vi "OE1022D_Configure Sensitivity and Filter.vi"(7 "OE1022D_Configure Sens and Filter":T1={"Dynamic Reserve"=1, "Sensitivity "=24, "Time Constant "=9, "Low Pass Filter Slope "=1, "Enable Sync Filter"=0, "Channel"=1} {"Channel" items=["A"=1, "B"=2]; "Enable Sync Filter" items=["OFF", "ON"]; "Low Pass Filter Slope" items=["6 dB/oct", "12 dB/oct", "18 db/oct", "24 dB/oct"]; "Time Constant" items=["10 us", "30 us", "100 us", "300 us", "1 ms", "3 ms", "10 ms", "30 ms", "100 ms", "300 ms", "1 s", "3 s", "10 s", "30 s", "100 s", "300 s", "1 ks", "3 ks"]; "Sensitivity" items=["1 nV/fA", "2 nV/fA", "5 nV/fA", "10 nV/fA", "20 nV/fA", "50 nV/fA", "100 nV/fA", "200 nV/fA", "500 nV/fA", "1 uV/pA", "2 uV/pA", "5 uV/pA", "10 uV/pA", "20 uV/pA", "50 uV/pA", "100 uV/pA", "200 uV/pA", "500 uV/pA", "1 mV/nA", "2 mV/nA", "5 mV/nA", "10 mV/nA", "20 mV/nA", "50 mV/nA", "100 mV/nA", "200 mV/nA", "500 mV/nA", "1 V/uA"]; "Dynamic Reserve" items=["Low Noise", "Normal", "High Reserve"]}, 8 "Error in (no error)":errorcluster caption="error out（no error）", 9 "Remote Mode":u16(ring) items=["USB", "RS232", "GPIB"], 11 "VISA resource name":refnum<visa-resource-name>) -> (0 "Error out":errorcluster caption="error out", 1 "Output String":string, 3 "VISA resource  out":refnum<visa-resource-name>)   [LabVIEW 2011]
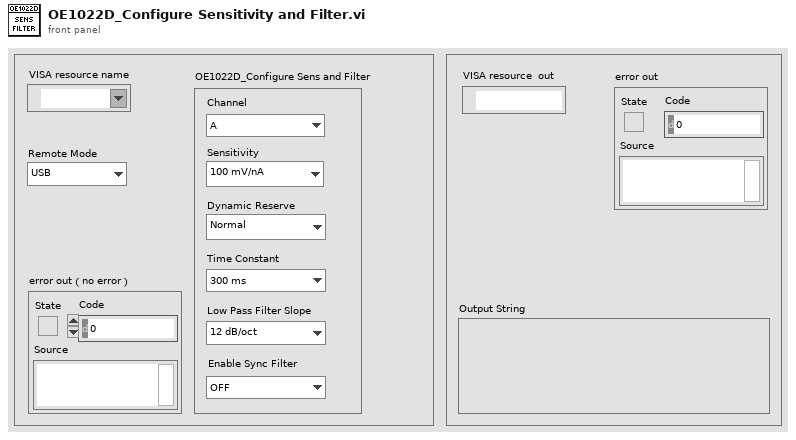
[diagram p1: front panel]
types:
  T1 = cluster{"Dynamic Reserve":u16, "Sensitivity ":u16, "Time Constant ":u8, "Low Pass Filter Slope ":u8, "Enable Sync Filter":u16, "Channel":u16}
  T2 = enum16{"ISRC", "IGND", "ICPL", "ILIN", "PHAS", "FMOD", "RSLP", "FREQ", "SWPT", "SLLM", "SULM", "SSLL", "SSLG", "STLM", "SWRM", "IRNG", "SENS", "RMOD", "OFLT", "OFSL", "SYNC", "DMOD", "HARM", "DARB", "SWVT", "SLVL", "SVLL", "SVUL", "SVSL", "SVSG", "SVTM", "SVRM", "RALL", "SNAP", "OUTP", "OAUX", "COUT", "CAUX", "COFP", "CEXP", "FPOP", "OEXP", "*IDN", "*RST", "OVLD", "INOV", "GNOV", "*PLL", "SSET", "RSET", "AGAN", "APHS", "ARSV", "ASCL", "EQCD", "EQCS", "SPED", "SRAT", "SLEN", "SSLE", "STRG", "SPRM", "STRD", "PAUS", "REST", "SPTS", "TRCA", "TEMP", "RSTU", "IHNZ", "DEQU", "SADD", "ARNG", "CSPE", "ISRCD", "IGNDD", "ICPLD", "ILIND", "PHASD", "FMODD", "RSLPD", "FREQD", "SWPTD", "SLLMD", "SULMD", "SSLLD", "SSLGD", "STLMD", "SWRMD", "SENSD", "RMODD", "OFLTD", "OFSLD", "SYNCD", "HARMD", "EQCDD", "EQCSD", "SNAPD", "OUTPD", "SWVTD", "SLVLD", "SVLLD", "SVULD", "SVSLD", "SVSGD", "SVTMD", "SVRMD", "SVDCD", "ARSVD", "AGAND", "APHSD", "ASCLD", "FPOPD", "CAUXD", "OEXPD", "SPEDD", "SRATD", "SLEND", "SSLED", "STRGD", "SPRMD", "STRDD", "PAUSD", "RESTD", "SPTSD", "TRCAD", "*IDND", "*RSTD", "INOVD", "GNOVD", "*PLLD", "SSETD", "RSETD"}
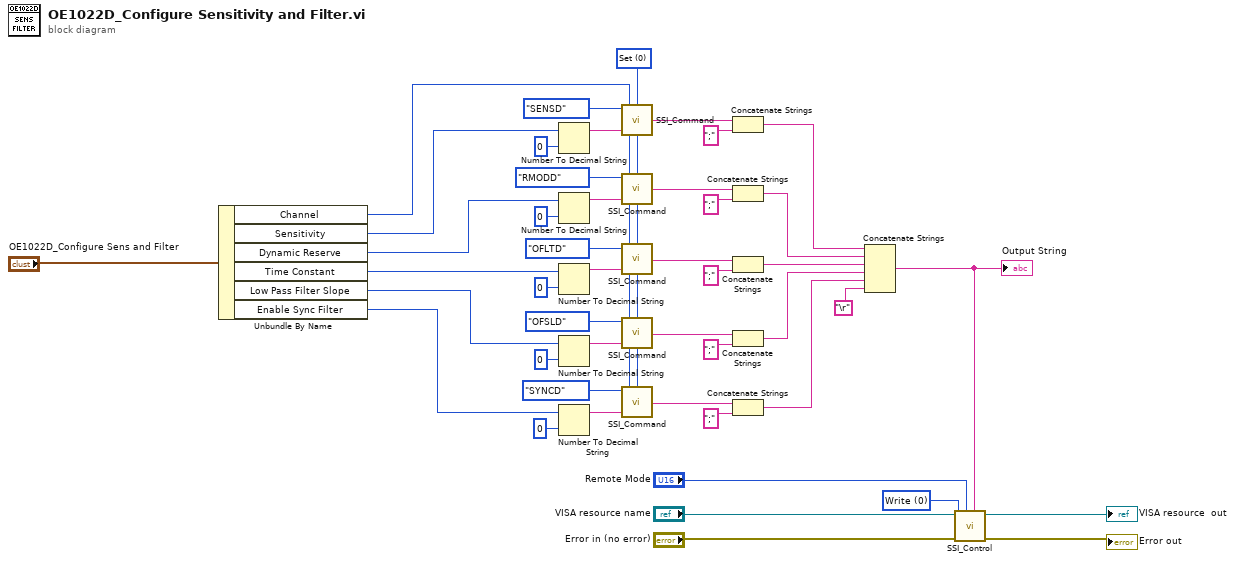
[diagram p0: block diagram]
diagram:
  w11 = u16 0 items=["Set", "Query"] ("Opera")
  w45 = u16 0 items=["Write", "Read"] ("Control")
  n1 = Unbundle By Name("OE1022D_Configure Sens and Filter") -> ("Channel"=w3:u16, "Sensitivity"=w21:u16, "Dynamic Reserve"=w20:u16, "Time Constant"=w19:u8, "Low Pass Filter Slope"=w18:u8, "Enable Sync Filter"=w10:u16)
  n2 = Number To Decimal String(number=w21, width (-)=i16 0 ("精度(6)")) -> (decimal integer string=w40:string)
  n3 = Number To Decimal String(number=w20, width (-)=i16 0 ("宽度(-)")) -> (decimal integer string=w38:string)
  n4 = Number To Decimal String(number=w19, width (-)=i16 0 ("宽度(-)")) -> (decimal integer string=w36:string)
  n5 = Number To Decimal String(number=w18, width (-)=i16 0 ("精度(6)")) -> (decimal integer string=w34:string)
  n6 = Number To Decimal String(number=w10, width (-)=i16 0 ("精度(6)")) -> (decimal integer string=w15:string)
  n7 = call "SSI_Command.vi"("Opera"=w11, "Paramter"=w40, "channel"=w3, "Command Type"=T2."SENSD") -> ("Output string"=w27:string)
  n8 = call "SSI_Command.vi"("Opera"=w11, "Paramter"=w38, "channel"=w3, "Command Type"=T2."RMODD") -> ("Output string"=w31:string)
  n9 = call "SSI_Command.vi"("Opera"=w11, "Paramter"=w36, "channel"=w3, "Command Type"=T2."OFLTD") -> ("Output string"=w25:string)
  n10 = call "SSI_Command.vi"("Opera"=w11, "Paramter"=w34, "channel"=w3, "Command Type"=T2."OFSLD") -> ("Output string"=w29:string)
  n11 = call "SSI_Command.vi"("Opera"=w11, "Paramter"=w15, "channel"=w3, "Command Type"=T2."SYNCD") -> ("Output string"=w12:string)
  n12 = Concatenate Strings(w27, ";" ("替换字符串(\"\")")) -> (w24:string)
  n13 = Concatenate Strings(w31, ";" ("替换字符串(\"\")")) -> (w23:string)
  n14 = Concatenate Strings(w25, ";" ("替换字符串(\"\")")) -> (w17:string)
  n15 = Concatenate Strings(w29, ";" ("替换字符串(\"\")")) -> (w16:string)
  n16 = Concatenate Strings(w12, ";" ("替换字符串(\"\")")) -> (w4:string)
  n17 = Concatenate Strings(w24, w23, w17, w16, w4, "\r") -> (w1:string)
  "Output String" <- w1
  n18 = call "SSI_Control.vi"("Write Buffer"=w1, "Remote Mode"="Remote Mode", "Error in (no error)"="Error in (no error)", "Control"=w45, "VISA resource name"="VISA resource name") -> ("Error out"=→"Error out":errorcluster, "VISA resource  out"=→"VISA resource  out":refnum<visa-resource-name>)  [unwired: 3 in, 2 out]
